vi "Analog Acq Cfg Popup.vi"(8 "error in (no error)":errorcluster, 11 "config file in":path caption="Configuration File") -> (0 "error out":errorcluster, 3 "config file out":path caption="Configuration File")   [LabVIEW 2022 SP3, in "Config Dialog.lvlib"]
uses:
  Config Dialog.lvlib
  <vilib>/Utility/miscctls.llb/LVPointTypeDef.ctl
  service/generation/controls/terminal configuration.ctl
  service/generation/controls/analog input settings.ctl
panel:
  in  "terminal configuration":T1 caption="Terminal configuration"
  in  "range":dbl=10.0 caption="Input range"
  out "output settings":T2={"sample rate"=0.0, "range"=0.0, "terminal configuration"=enum."Pseudodifferential"}
  in  "Save":bool
  in  "sample rate":dbl=25600.0 caption="Sampling rate" format="%#_6pS/s"
  # "Analog Input Configuration"
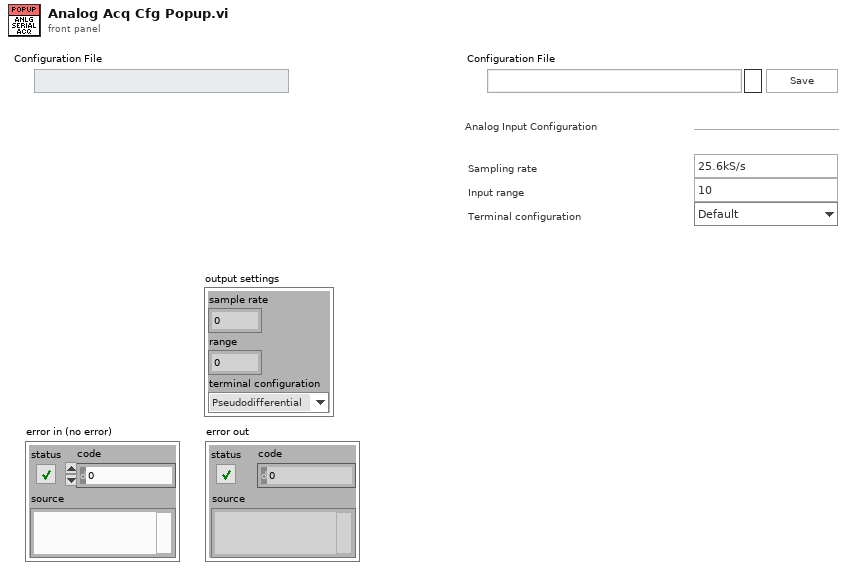
[diagram p1: front panel]
types:
  T1 = typedef "AudioGenTypeDefs.lvlib/terminal configuration.ctl" = enum32{"Default", "RSE", "Differential", "Pseudodifferential"}
  T2 = typedef "AudioGenTypeDefs.lvlib/analog input settings.ctl" = cluster{"sample rate":dbl, "range":dbl, "terminal configuration":T1}
  T3 = typedef "LVPointTypeDef.ctl" = cluster{"Horizontal":i16, "Vertical":i16}
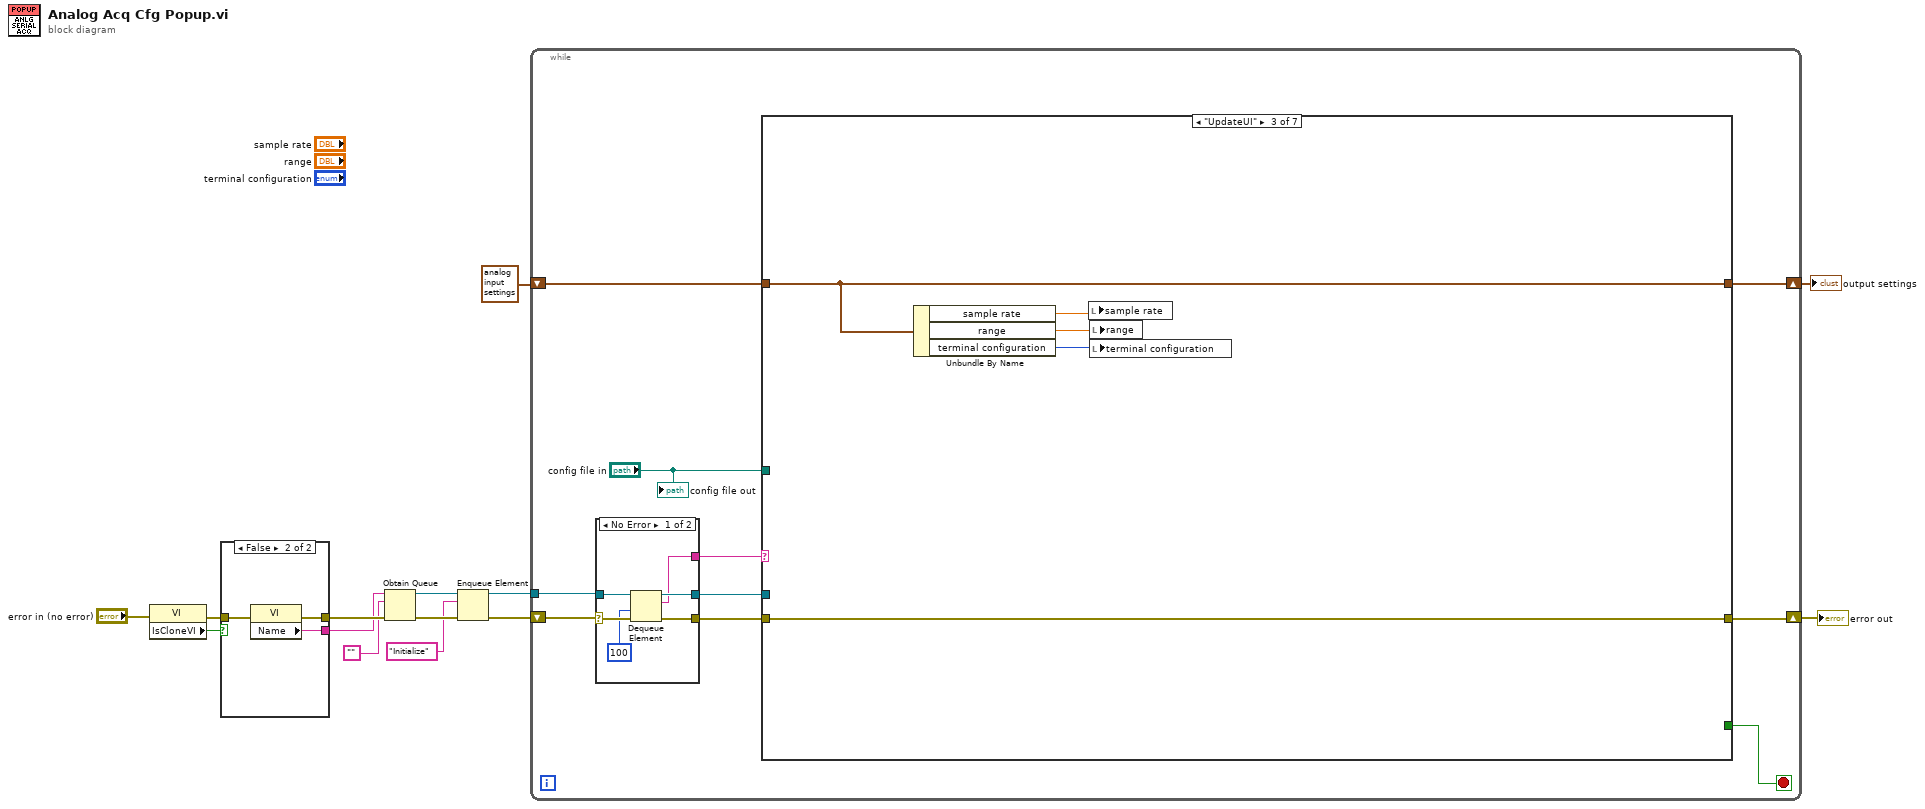
[diagram p0: block diagram]
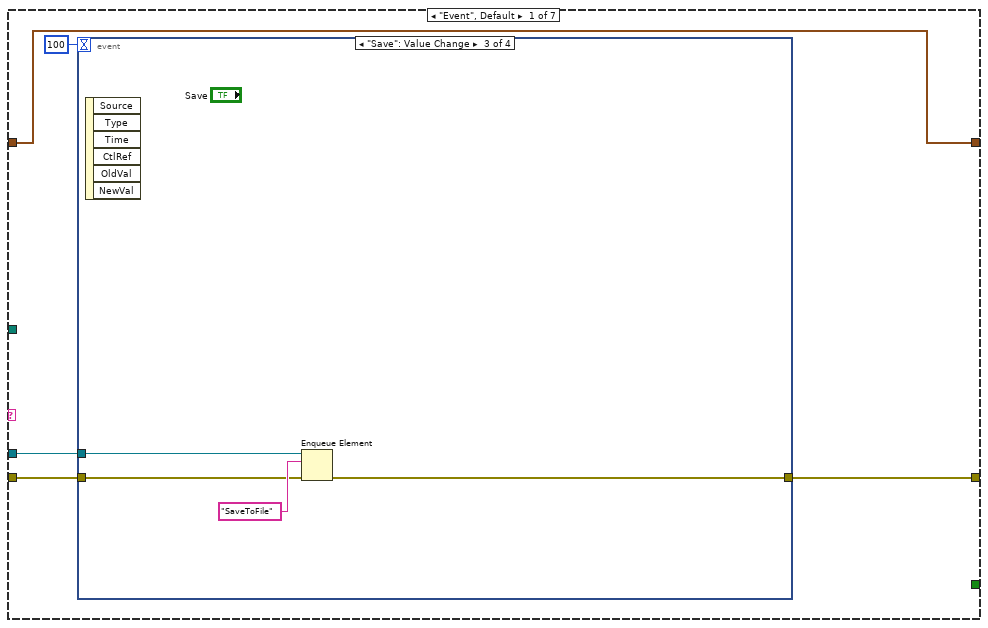
[diagram p2: hidden frame]
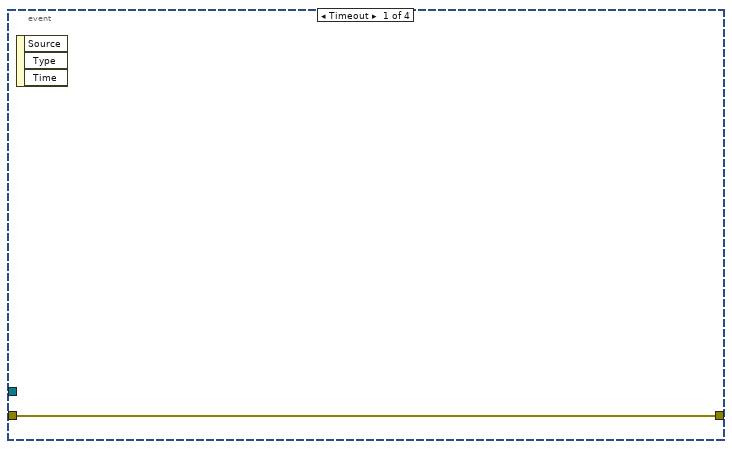
[diagram p3: hidden frame]
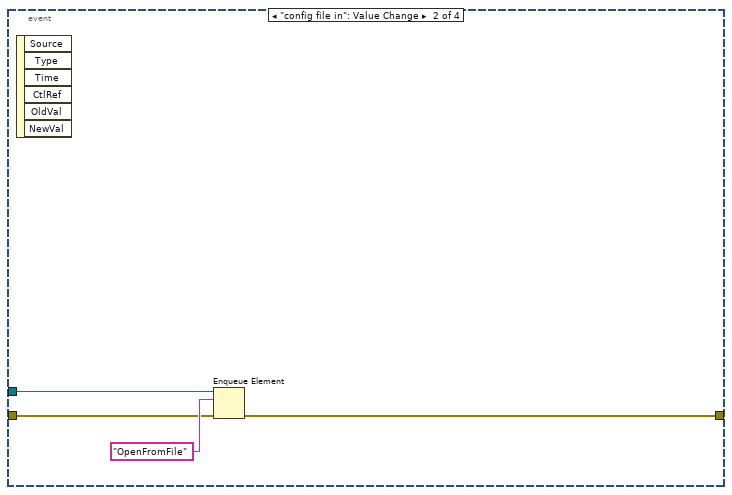
[diagram p4: hidden frame]
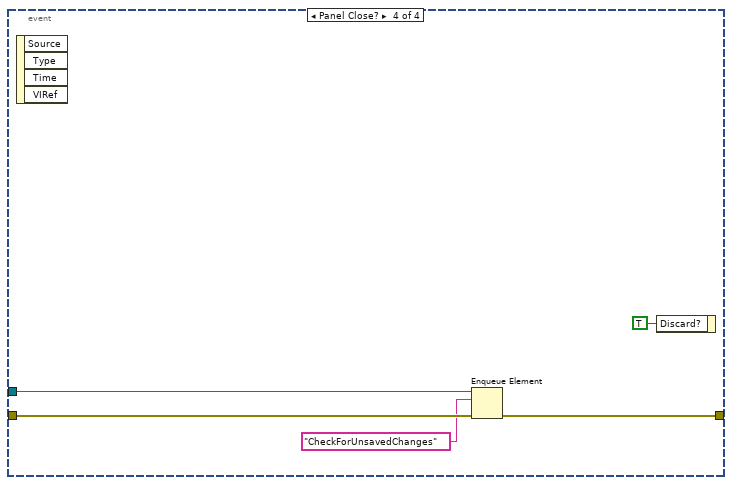
[diagram p5: hidden frame]
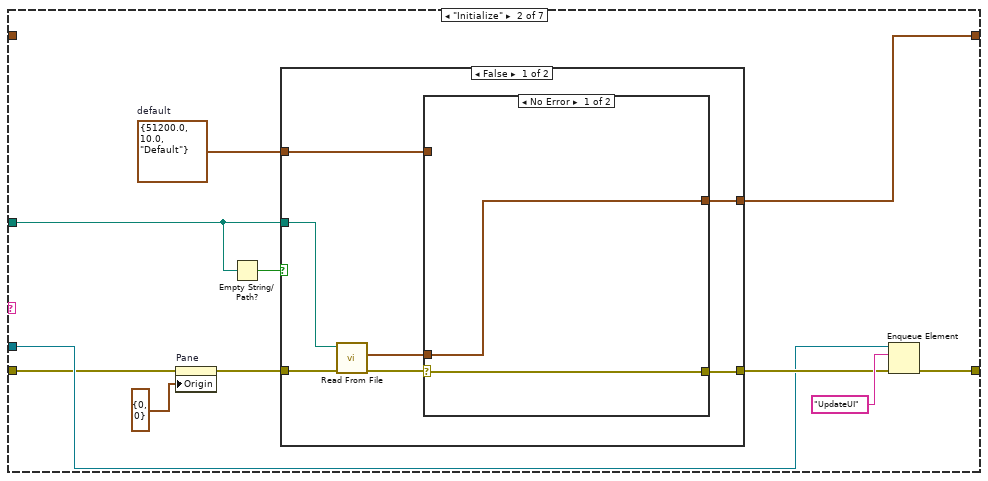
[diagram p6: hidden frame]
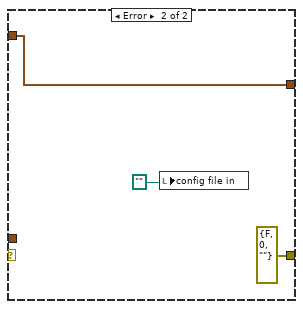
[diagram p7: hidden frame]
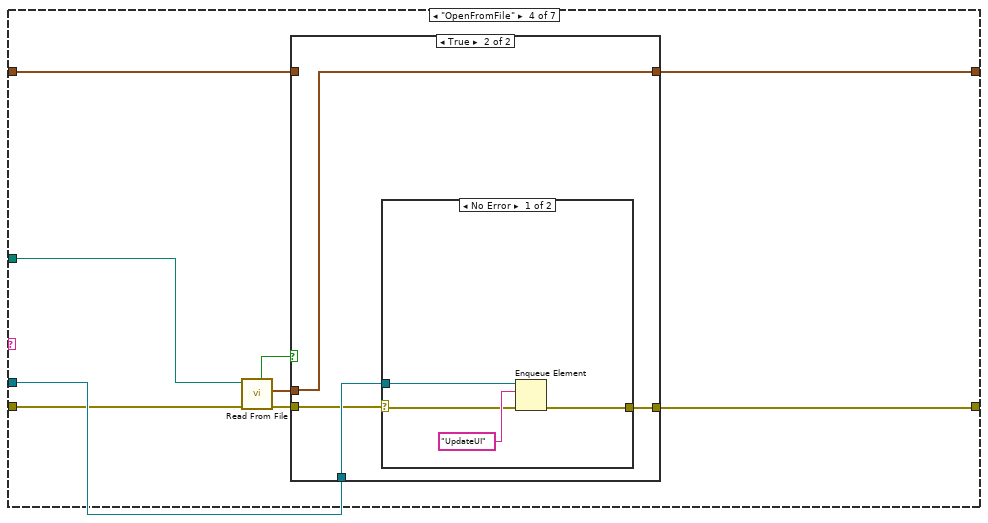
[diagram p9: hidden frame]
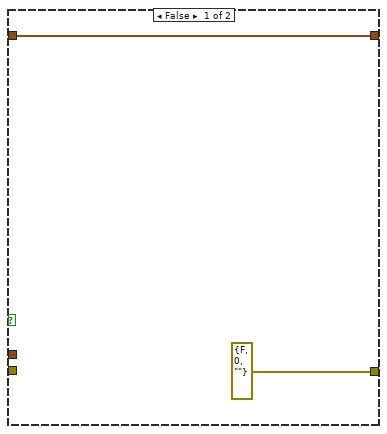
[diagram p10: hidden frame]
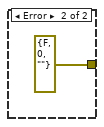
[diagram p11: hidden frame]
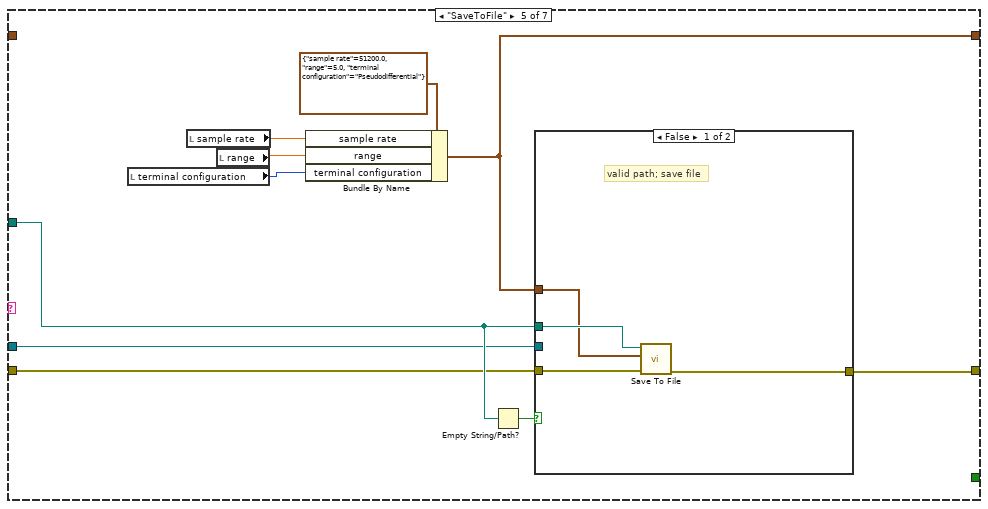
[diagram p12: hidden frame]
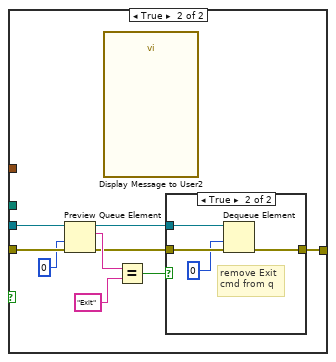
[diagram p13: hidden frame]
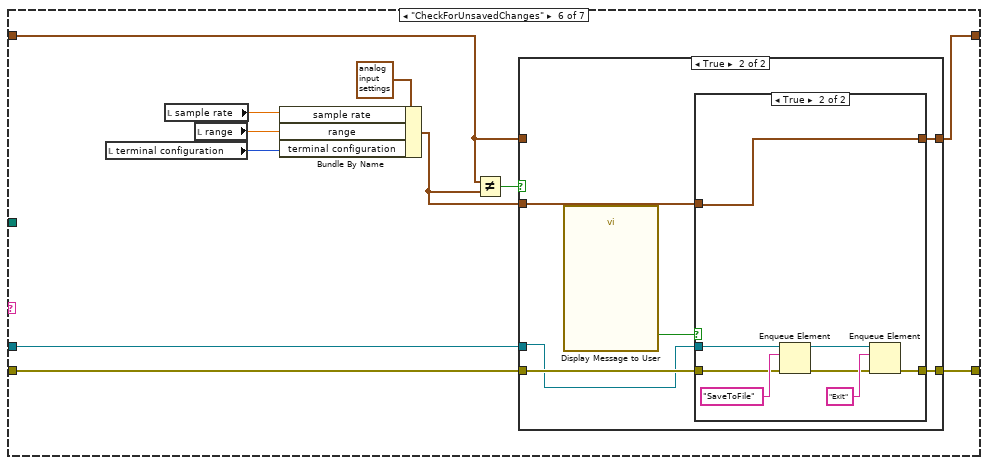
[diagram p15: hidden frame]
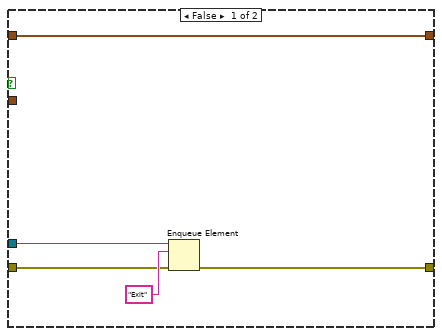
[diagram p16: hidden frame]
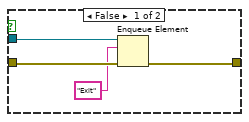
[diagram p17: hidden frame]
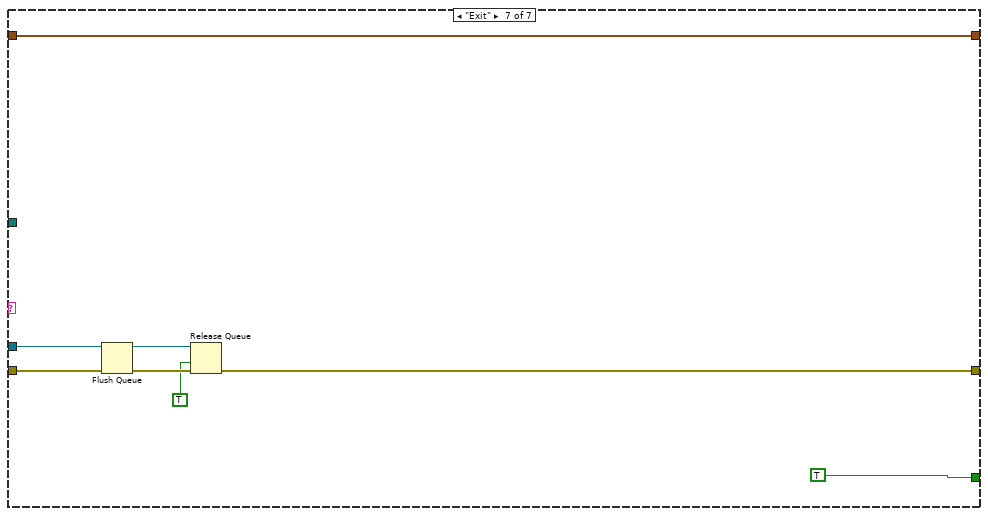
[diagram p18: hidden frame]
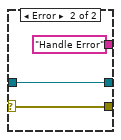
[diagram p19: hidden frame]
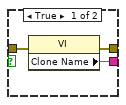
[diagram p20: hidden frame]
diagram:
  n1 = property class="VI"(error in="error in (no error)") -> (error out=w7:errorcluster, "IsCloneVI"=w8:bool)  [unwired: 1 in, 1 out]
  n2 = case shown="False" w8 {
    tunnel: [w17 w20] -> w14
    tunnel: [w16 w19] -> w13
    tunnel: w7 -> [w15 w18]
    frame True {
      n3 = property class="VI"(error in=w15) -> (error out=w17:errorcluster, "Clone Name"=w16:string)  [unwired: 1 in, 1 out]
    }
    frame False {
      n4 = property class="VI"(error in=w18) -> (error out=w20:errorcluster, "Name"=w19:string)  [unwired: 1 in, 1 out]
    }
  }
  n5 = Obtain Queue(name (unnamed)=w13, element data type="", error in (no error)=w14) -> (queue out=w11:refnum<queue>, error out=w12:errorcluster)  [unwired: 2 in, 1 out]
  n6 = Enqueue Element(queue=w11, element="Initialize", error in (no error)=w12) -> (queue out=w5:refnum<queue>, error out=w6:errorcluster)  [unwired: 1 in, 1 out]
  n7 = while {
    tunnel: w5 -> [w29]
    shift-right: [w25] -> w4
    shift-left: w6 -> [w30]
    shift-right: [w22] -> w1
    shift-left: T2 {"sample rate"=51200.0, "range"=5.0, "terminal configuration"=enum."Pseudodifferential"} ("output settings") -> [w23]
    stop <- w24 stop-if-true
    n8 = case shown="No Error" w30 {
      selector: w30 -> [w175 w178]
      tunnel: [w174 w178] -> w26
      tunnel: w29 -> [w173 w177]
      tunnel: [w172 w177] -> w27
      tunnel: [w171 "Handle Error"] -> w28
      frame No Error {
        n9 = Dequeue Element(queue=w173, timeout in ms (-1)=100, error in (no error)=w175) -> (queue out=w172:refnum<queue>, element=w171:string, error out=w174:errorcluster)  [unwired: 1 out]
      }
      frame Error {
      }
    }
    n10 = case shown="\"UpdateUI\"" w28 {
      tunnel: w27 -> [w33 w54 _ w88 w104 w134 w165]
      tunnel: w26 -> [w34 w52 w79 w85 w106 w137 w166]
      tunnel: [w32 w55 w79 w87 w109 w136 w163] -> w25
      tunnel: [_ _ _ _ _ _ TRUE] -> w24
      tunnel: w23 -> [w31 _ w78 w82 _ w132 w162]
      tunnel: [w31 w58 w78 w81 w108 w135 w162] -> w22
      tunnel: "config file in" -> [_ w59 _ w86 w107 _ _]
      frame "Event", Default {
        n11 = event shown="[2] \"Save\": Value Change" {
          selector: _ -> [_ _ _ _]
          dyn-events: _ -> [_ _ _ _]
          timeout: 100 -> [_ _ _ _]
          tunnel: w34 -> [w36 w39 w43 w48]
          tunnel: w33 -> [_ w38 w42 w47]
          tunnel: [w36 w37 w41 w46] -> w32
          event Timeout {
            n12 = event-data() -> ()  [unwired: 1 in, 3 out]
          }
          event "config file in": Value Change {
            n13 = event-data() -> ()  [unwired: 1 in, 6 out]
            n14 = Enqueue Element(queue=w38, element="OpenFromFile", error in (no error)=w39) -> (error out=w37:errorcluster)  [unwired: 1 in, 2 out]
          }
          event "Save": Value Change {
            n15 = event-data() -> ()  [unwired: 1 in, 6 out]
            n16 = Enqueue Element(queue=w42, element="SaveToFile", error in (no error)=w43) -> (error out=w41:errorcluster)  [unwired: 1 in, 2 out]
          }
          event Panel Close? {
            n17 = event-data() -> ()  [unwired: 1 in, 4 out]
            n18 = Enqueue Element(queue=w47, element="CheckForUnsavedChanges", error in (no error)=w48) -> (error out=w46:errorcluster)  [unwired: 1 in, 2 out]
            n19 = event-data("Discard?"=TRUE) -> ()  [unwired: 1 in, 1 out]
          }
        }
      }
      frame "Initialize" {
        w50 = T2 {"sample rate"=51200.0, "range"=10.0, "terminal configuration"=enum."Default"}  # default
        n20 = property on="Pane" class="Pane"(error in=w52, "Origin"=T3 {"Horizontal"=0, "Vertical"=0}) -> (error out=w51:errorcluster)  [unwired: 1 in, 1 out]
        n21 = Empty String/Path?(string/path=w59) -> (empty?=w60:bool)
        n22 = case shown="False" w60 {
          tunnel: w51 -> [w67 w74]
          tunnel: w59 -> [w66 _]
          tunnel: [w61 w73] -> w58
          tunnel: [w63 w74] -> w56
          tunnel: w50 -> [w62 w73]
          frame False {
            n23 = call "Read From File.vi"("error in (no error)"=w67, "file path"=w66) -> ("error out"=w65:errorcluster, "analog input"=w64:T2)  [unwired: 7 in, 1 out]
            n24 = case shown="No Error" w65 {
              selector: w65 -> [w68 _]
              tunnel: w64 -> [w69 _]
              tunnel: [w69 w70] -> w61
              tunnel: [w68 errorcluster {"status"=FALSE, "code"=0, "source"=""} ("error IO")] -> w63
              tunnel: w62 -> [_ w70]
              frame No Error {
              }
              frame Error {
                n25 = local write "config file in"(path "") -> ()
              }
            }
          }
          frame True {
          }
        }
        n26 = Enqueue Element(queue=w54, element="UpdateUI", error in (no error)=w56) -> (error out=w55:errorcluster)  [unwired: 1 in, 2 out]
      }
      frame "UpdateUI" {
        n27 = Unbundle By Name(w78) -> ("sample rate"=w77:dbl, "range"=w76:dbl, "terminal configuration"=w75:T1)
        n28 = local write "sample rate"(w77) -> ()
        n29 = local write "range"(w76) -> ()
        n30 = local write "terminal configuration"(w75) -> ()
      }
      frame "OpenFromFile" {
        n31 = call "Read From File.vi"("error in (no error)"=w85, "file path"=w86) -> ("error out"=w84:errorcluster, "analog input"=w80:T2, "file exists?"=w83:bool)  [unwired: 7 in]
        n32 = case shown="True" w83 {
          tunnel: w88 -> [_ w94]
          tunnel: [errorcluster {"status"=FALSE, "code"=0, "source"=""} ("error out") w93] -> w87
          tunnel: w84 -> [_ w91]
          tunnel: w82 -> [w90 _]
          tunnel: [w90 w92] -> w81
          tunnel: w80 -> [_ w92]
          frame False {
          }
          frame True {
            n33 = case shown="No Error" w91 {
              selector: w91 -> [w95 _]
              tunnel: w94 -> [w97 _]
              tunnel: [w96 errorcluster {"status"=FALSE, "code"=0, "source"=""} ("error out")] -> w93
              frame No Error {
                n34 = Enqueue Element(queue=w97, element="UpdateUI", error in (no error)=w95) -> (error out=w96:errorcluster)  [unwired: 1 in, 2 out]
              }
              frame Error {
              }
            }
          }
        }
      }
      frame "SaveToFile" {
        n35 = local read "terminal configuration"() -> (w100:T1)
        n36 = local read "sample rate"() -> (w102:dbl)
        n37 = local read "range"() -> (w101:dbl)
        n38 = Bundle By Name(cluster=T2 {"sample rate"=51200.0, "range"=5.0, "terminal configuration"=enum."Pseudodifferential"} ("output settings"), "sample rate"=w102, "range"=w101, "terminal configuration"=w100) -> (w108:T2)
        n39 = Empty String/Path?(string/path=w107) -> (empty?=w105:bool)
        n40 = case shown="False" w105 {
          tunnel: [w113 w115] -> w109
          tunnel: w108 -> [w110 _]
          tunnel: w107 -> [w112 _]
          tunnel: w106 -> [w111 w122]
          tunnel: w104 -> [_ w121]
          frame False {
            # "valid path; save file"
            n41 = call "Save To File.vi"("error in (no error)"=w111, "output settings"=w110, "file path"=w112) -> ("error out"=w113:errorcluster)  [unwired: 8 in]
          }
          frame True {
            n42 = Preview Queue Element(queue=w121, timeout in ms (-1)=0, error in (no error)=w122) -> (queue out=w118:refnum<queue>, element=w120:string, error out=w116:errorcluster)  [unwired: 1 out]
            n43 = call "Display Message to User2"() -> ()  [unwired: 10 in, 2 out]
            n44 = Equal?(x=w120, y="Exit") -> (x = y?=w117:bool)
            n45 = case shown="True" w117 {
              tunnel: w118 -> [_ w127]
              tunnel: w116 -> [w123 w126]
              tunnel: [w123 w125] -> w115
              frame False {
              }
              frame True {
                # "remove Exit\ncmd from q"
                n46 = Dequeue Element(queue=w127, timeout in ms (-1)=0, error in (no error)=w126) -> (error out=w125:errorcluster)  [unwired: 3 out]
              }
            }
          }
        }
      }
      frame "CheckForUnsavedChanges" {
        n47 = local read "terminal configuration"() -> (w130:T1)
        n48 = local read "sample rate"() -> (w128:dbl)
        n49 = local read "range"() -> (w129:dbl)
        n50 = Bundle By Name(cluster=T2 {"sample rate"=51200.0, "range"=5.0, "terminal configuration"=enum."Pseudodifferential"} ("output settings"), "sample rate"=w128, "range"=w129, "terminal configuration"=w130) -> (w133:T2)
        n51 = Not Equal?(x=w132, y=w133) -> (x != y?=w138:bool)
        n52 = case shown="True" w138 {
          tunnel: w137 -> [w141 w149]
          tunnel: [w139 w145] -> w136
          tunnel: w133 -> [_ w147]
          tunnel: w132 -> [w143 _]
          tunnel: [w143 w146] -> w135
          tunnel: w134 -> [w140 w144]
          frame False {
            n53 = Enqueue Element(queue=w140, element="Exit", error in (no error)=w141) -> (error out=w139:errorcluster)  [unwired: 1 in, 2 out]
          }
          frame True {
            n54 = call "Display Message to User"() -> ("Yes"=w148:bool)  [unwired: 10 in, 1 out]
            n55 = case shown="True" w148 {
              tunnel: w149 -> [w153 w160]
              tunnel: w147 -> [_ w159]
              tunnel: [_ w159] -> w146
              tunnel: [w151 w155] -> w145
              tunnel: w144 -> [w152 w154]
              frame False {
                n56 = Enqueue Element(queue=w152, element="Exit", error in (no error)=w153) -> (error out=w151:errorcluster)  [unwired: 1 in, 2 out]
              }
              frame True {
                n57 = Enqueue Element(queue=w154, element="SaveToFile", error in (no error)=w160) -> (queue out=w156:refnum<queue>, error out=w157:errorcluster)  [unwired: 1 in, 1 out]
                n58 = Enqueue Element(queue=w156, element="Exit", error in (no error)=w157) -> (error out=w155:errorcluster)  [unwired: 1 in, 2 out]
              }
            }
          }
        }
      }
      frame "Exit" {
        n59 = Flush Queue(queue=w165, error in (no error)=w166) -> (queue out=w169:refnum<queue>, error out=w168:errorcluster)  [unwired: 1 out]
        n60 = Release Queue(queue=w169, force destroy? (F)=TRUE, error in (no error)=w168) -> (error out=w163:errorcluster)  [unwired: 2 out]
      }
    }
    "config file out" <- "config file in"
  }
  "error out" <- w4
  "output settings" <- w1
